vi "Settings Dialog.vi"(8 "error in (no error)":errorcluster, 11 "Settings in":T5={"Acquisition"={"State"=enum."Idle S3DK", "Settings"="", "Online"=FALSE, "S3DK"={"Signals"={"Phasor"=[], "Analog"=[], "Digital"=[]}}, "CSV"={"CSV Path"=path "", "Index"=0, "Parcel Length"=0, "EOF?"=FALSE}}, "Logging"={"Logging State"=enum."Idle", "Settings"="", "Buffer"={"Index"=0, "Size"=15000, "Samples"=0, "Ordered ?"=FALSE}}, "Processing"={"Settings"="Processing", "Params Energy"={"Index"=0, "Size"=0, "Samples"=0, "Ordered ?"=FALSE}, "Refresh Rate"=0, "Filters Instances"=[], "Levels"={"Low"=0, "High"=0, "Danger"=0}, "Params PSD"={"Index"=0, "Size"=0, "Samples"=0, "Ordered ?"=FALSE}, "PSD Instances"=[], "Filter Config"=[], "PSDs"=[]}} {"Processing"."PSD Instances"."Averaging"."averaging mode" items=["No averaging", "RMS averaging", "Peak hold"]; "Processing"."PSD Instances"."Averaging"."weighting mode" items=["Linear", "Exponential"]; "Processing"."PSD Instances"."AR"."Method" items=["Forward-Backward", "Least-Squares", "Yule-Walker", "Burg-Lattice", "Geometric-Lattice"]; "Processing"."PSD Instances"."Welch"."window info"."window" items=["None ", "Hanning", "Hamming", "Blackman-Harris", "Exact Blackman", "Blackman", "Flat Top", "4 Term B-Harris ", "7 Term B-Harris", "Low Sidelobe"]; "Processing"."Filters Instances"."PSD Filter"."Forward Coefficients" format="%.4f"; "Processing"."Filters Instances"."PSD Filter"."Reverse Coefficients" format="%.4f"}) -> (0 "error out":errorcluster, 1 "Changed?":bool, 2 "UI Refresh Needed?":bool, 3 "Settings out":T5={"Acquisition"={"State"=enum."Idle S3DK", "Settings"="", "Online"=FALSE, "S3DK"={"Signals"={"Phasor"=[], "Analog"=[], "Digital"=[]}}, "CSV"={"CSV Path"=path "", "Index"=0, "Parcel Length"=0, "EOF?"=FALSE}}, "Logging"={"Logging State"=enum."Idle", "Settings"="", "Buffer"={"Index"=0, "Size"=15000, "Samples"=0, "Ordered ?"=FALSE}}, "Processing"={"Settings"="Processing", "Params Energy"={"Index"=0, "Size"=0, "Samples"=0, "Ordered ?"=FALSE}, "Refresh Rate"=0, "Filters Instances"=[], "Levels"={"Low"=0, "High"=0, "Danger"=0}, "Params PSD"={"Index"=0, "Size"=0, "Samples"=0, "Ordered ?"=FALSE}, "PSD Instances"=[], "Filter Config"=[], "PSDs"=[]}} {"Processing"."PSD Instances"."Averaging"."averaging mode" items=["No averaging", "RMS averaging", "Peak hold"]; "Processing"."PSD Instances"."Averaging"."weighting mode" items=["Linear", "Exponential"]; "Processing"."PSD Instances"."AR"."Method" items=["Forward-Backward", "Least-Squares", "Yule-Walker", "Burg-Lattice", "Geometric-Lattice"]; "Processing"."PSD Instances"."Welch"."window info"."window" items=["None ", "Hanning", "Hamming", "Blackman-Harris", "Exact Blackman", "Blackman", "Flat Top", "4 Term B-Harris ", "7 Term B-Harris", "Low Sidelobe"]; "Processing"."Filters Instances"."PSD Filter"."Forward Coefficients" format="%.4f"; "Processing"."Filters Instances"."PSD Filter"."Reverse Coefficients" format="%.4f"})   [LabVIEW 2017, in "Settings.lvlib"]
doc: "Dialog for selecting user specified settings."
uses:
  Settings.lvlib
  Settings.ctl
  acquisition/Acquisition Settings.ctl
  acquisition/Acquisition State.ctl
  logging/Logging Configuration.ctl
  logging/Logging State.ctl
  libs/PMU Buffer/Buffer Settings.ctl
  processing/Processing Settings.ctl
  processing/Filters.ctl
  processing/Levels.ctl
  processing/PSD Setting.ctl
  processing/BP Filter Settings.ctl
  <vilib>/Analysis/3filter.llb/Filter Passband Type.ctl
  acquisition/Acquisition.lvlib
  logging/Logging.lvlib
  processing/Processing.lvlib
  libs/PMU Buffer/PMU data buffer.lvlib
  <vilib>/Analysis/NI_AALBase.lvlib
panel:
  in  "Levels":T1
  in  "Tab Control":T2(tab)
  in  "Set 1":T3 {"Averaging"."Nb" min=1; "Averaging"."Weighting Mode" items=["Linear", "Exponential"]; "Averaging"."Averaging Mode" items=["No averaging", "RMS averaging", "Peak hold"]; "Welch"."window info"."window" items=["None ", "Hanning", "Hamming", "Blackman-Harris", "Exact Blackman", "Blackman", "Flat Top", "4 Term B-Harris ", "7 Term B-Harris", "Low Sidelobe"]; "AR"."Method" items=["Forward-Backward", "Least-Squares", "Yule-Walker", "Burg-Lattice", "Geometric-Lattice"]}
  in  "Set 1":T4={"Type"=enum."Bandpass", "Freq low"=0.11, "Freq high"=1.0, "Filter Order"=11} {"Filter Order" min=2 max=15 scale=7.0..15.0}
  in  "Set 2":T4={"Type"=enum."Bandpass", "Freq low"=0.11, "Freq high"=1.0, "Filter Order"=11} {"Filter Order" min=2 max=15 scale=7.0..15.0}
  in  "Set 2":T3 {"Averaging"."Nb" min=1; "Averaging"."Weighting Mode" items=["Linear", "Exponential"]; "Averaging"."Averaging Mode" items=["No averaging", "RMS averaging", "Peak hold"]; "Welch"."window info"."window" items=["None ", "Hanning", "Hamming", "Blackman-Harris", "Exact Blackman", "Blackman", "Flat Top", "4 Term B-Harris ", "7 Term B-Harris", "Low Sidelobe"]; "AR"."Method" items=["Forward-Backward", "Least-Squares", "Yule-Walker", "Burg-Lattice", "Geometric-Lattice"]}
  in  "Set 3":T4={"Type"=enum."Bandpass", "Freq low"=0.11, "Freq high"=1.0, "Filter Order"=11} {"Filter Order" min=2 max=15 scale=7.0..15.0}
  in  "Set 3":T3 {"Averaging"."Nb" min=1; "Averaging"."Weighting Mode" items=["Linear", "Exponential"]; "Averaging"."Averaging Mode" items=["No averaging", "RMS averaging", "Peak hold"]; "Welch"."window info"."window" items=["None ", "Hanning", "Hamming", "Blackman-Harris", "Exact Blackman", "Blackman", "Flat Top", "4 Term B-Harris ", "7 Term B-Harris", "Low Sidelobe"]; "AR"."Method" items=["Forward-Backward", "Least-Squares", "Yule-Walker", "Burg-Lattice", "Geometric-Lattice"]}
  in  "Set 4":T4={"Type"=enum."Bandpass", "Freq low"=0.11, "Freq high"=1.0, "Filter Order"=11} {"Filter Order" min=2 max=15 scale=7.0..15.0}
  in  "Set 4":T3 {"Averaging"."Nb" min=1; "Averaging"."Weighting Mode" items=["Linear", "Exponential"]; "Averaging"."Averaging Mode" items=["No averaging", "RMS averaging", "Peak hold"]; "Welch"."window info"."window" items=["None ", "Hanning", "Hamming", "Blackman-Harris", "Exact Blackman", "Blackman", "Flat Top", "4 Term B-Harris ", "7 Term B-Harris", "Low Sidelobe"]; "AR"."Method" items=["Forward-Backward", "Least-Squares", "Yule-Walker", "Burg-Lattice", "Geometric-Lattice"]}
  in  "Online?":bool
  in  "Parcel Length":i32
  in  "Path":path
  in  "Refresh Rate":u32(ring) caption="Hz" items=["1"=1000, "5"=200, "10"=100, "25"=40, "50"=20]
  in  "Buffer Size":i32
  in  "Cancel Button":bool
  in  "OK Button":bool
  # "Non visible portion of dialog (needed for connector pane)."
  # "Welch Parameter"
  # "AR Spectrum"
  # "Welch Parameter"
  # "AR Spectrum"
  # "Welch Parameter"
  # "AR Spectrum"
  # "Welch Parameter"
  # "AR Spectrum"
  # "Buffer Paremeters"
  # "Buffer Paremeters"
  # "Buffer Paremeters"
  # "Buffer Paremeters"
  # "Buffer Paremeters"
  # "Buffer Paremeters"
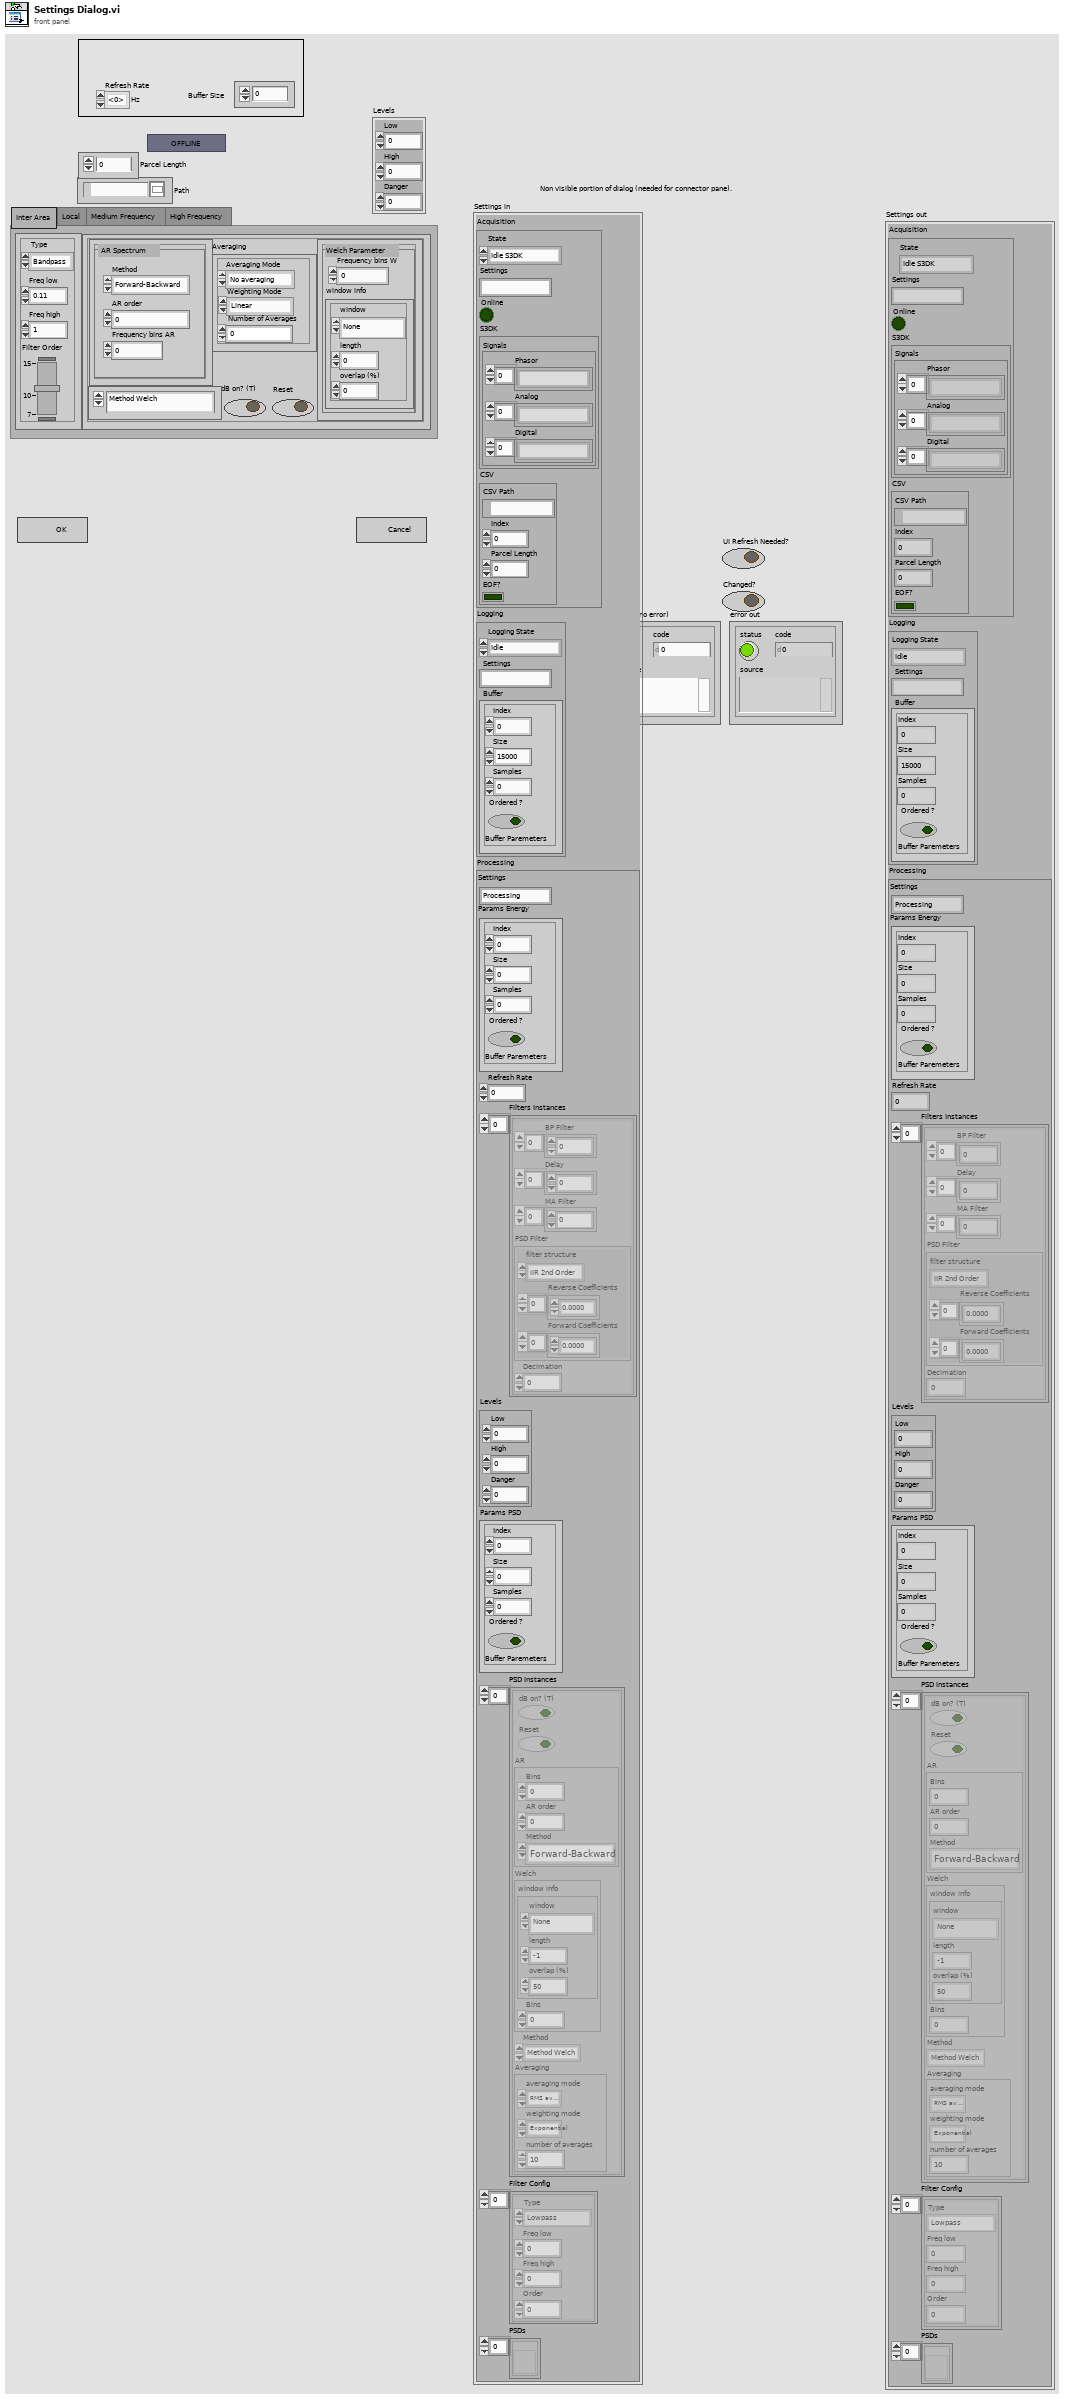
[diagram p1: front panel]
types:
  T1 = typedef "Processing.lvlib/Levels.ctl" = cluster{"Low":i32, "High":i32, "Danger":i32}
  T2 = enum32{"Inter Area", "Local", "Medium Frequency", "High Frequency"}
  T3 = cluster{"dB on? (T)":bool, "Reset":bool, "AR":cluster{"Bins":i32, "Method":u16, "AR order":i32}, "Welch":cluster{"window info":cluster{"window":u16, "length":i32, "overlap (%)":dbl}, "Bins":i32}, "Method":enum16{"Method Welch", "Method AR", "Both"}, "Averaging":cluster{"Averaging Mode":u16, "Weighting Mode":u16, "Nb":u32}}
  T4 = cluster{"Type":enum16{"Lowpass", "Highpass", "Bandpass", "Bandstop"}, "Freq low":dbl, "Freq high":dbl, "Filter Order":i32}
  T5 = typedef "Settings.lvlib/Settings.ctl" = cluster{"Acquisition":T6, "Logging":T8, "Processing":T11}
  T6 = typedef "Acquisition.lvlib/Acquisition Settings.ctl" = cluster{"State":T7, "Settings":string, "Online":bool, "S3DK":cluster{"Signals":cluster{"Phasor":string[], "Analog":string[], "Digital":string[]}}, "CSV":cluster{"CSV Path":path, "Index":i32, "Parcel Length":i32, "EOF?":bool}}
  T7 = typedef "Acquisition.lvlib/Acquisition State.ctl" = enum16{"Idle", "Idle S3DK", "Acquiring S3DK", "Idle CSV", "Acquiring CSV"}
  T8 = typedef "Logging.lvlib/Logging Configuration.ctl" = cluster{"Logging State":T9, "Settings":string, "Buffer":T10}
  T9 = typedef "Logging.lvlib/Logging State.ctl" = enum16{"Idle", "Logging"}
  T10 = typedef "PMU data buffer.lvlib/Buffer Settings.ctl" = cluster{"Index":i32, "Size":i32, "Samples":i32, "Ordered ?":bool}
  T11 = typedef "Processing.lvlib/Processing Settings.ctl" = cluster{"Settings":string, "Params Energy":T10, "Refresh Rate":u32, "Filters Instances":T12[], "Levels":T1, "Params PSD":T10, "PSD Instances":T13[], "Filter Config":T14[], "PSDs":refnum<vi>[]}
  T12 = typedef "Processing.lvlib/Filters.ctl" = cluster{"BP Filter":dbl[], "Delay":dbl[], "MA Filter":dbl[], "PSD Filter":cluster{"filter structure":enum32{"IIR 2nd Order", "IIR 4th Order"}, "Reverse Coefficients":dbl[], "Forward Coefficients":dbl[]}, "Decimation":i32}
  T13 = typedef "Processing.lvlib/PSD Setting.ctl" = cluster{"dB on? (T)":bool, "Reset":bool, "AR":cluster{"Bins":i32, "AR order":i32, "Method":u16}, "Welch":cluster{"window info":cluster{"window":u16, "length":i32, "overlap (%)":dbl}, "Bins":i32}, "Method":enum16{"Method Welch", "Method AR", "Both"}, "Averaging":cluster{"averaging mode":u16, "weighting mode":u16, "number of averages":u32}}
  T14 = typedef "Processing.lvlib/BP Filter Settings.ctl" = cluster{"Type":T15, "Freq low":dbl, "Freq high":dbl, "Order":i32}
  T15 = typedef "NI_AALBase.lvlib/Filter Passband Type.ctl" = enum32{"Lowpass", "Highpass", "Bandpass", "Bandstop"}
  T16 = cluster{"dB on? (T)":bool, "Reset":bool, "AR":cluster{"Bins":i32, "Method":u16, "AR order":i32}, "Welch":cluster{"window info":cluster{"window":u16, "length":i32, "overlap (%)":dbl}, "Bins":i32}, "Method":enum16{"Method Welch", "Method AR", "Both"}, "Averaging":cluster{"Averaging Mode":u16, "Weighting Mode":u16, "Nb":u32}}[]
  T17 = cluster{"Type":enum16{"Lowpass", "Highpass", "Bandpass", "Bandstop"}, "Freq low":dbl, "Freq high":dbl, "Filter Order":i32}[]
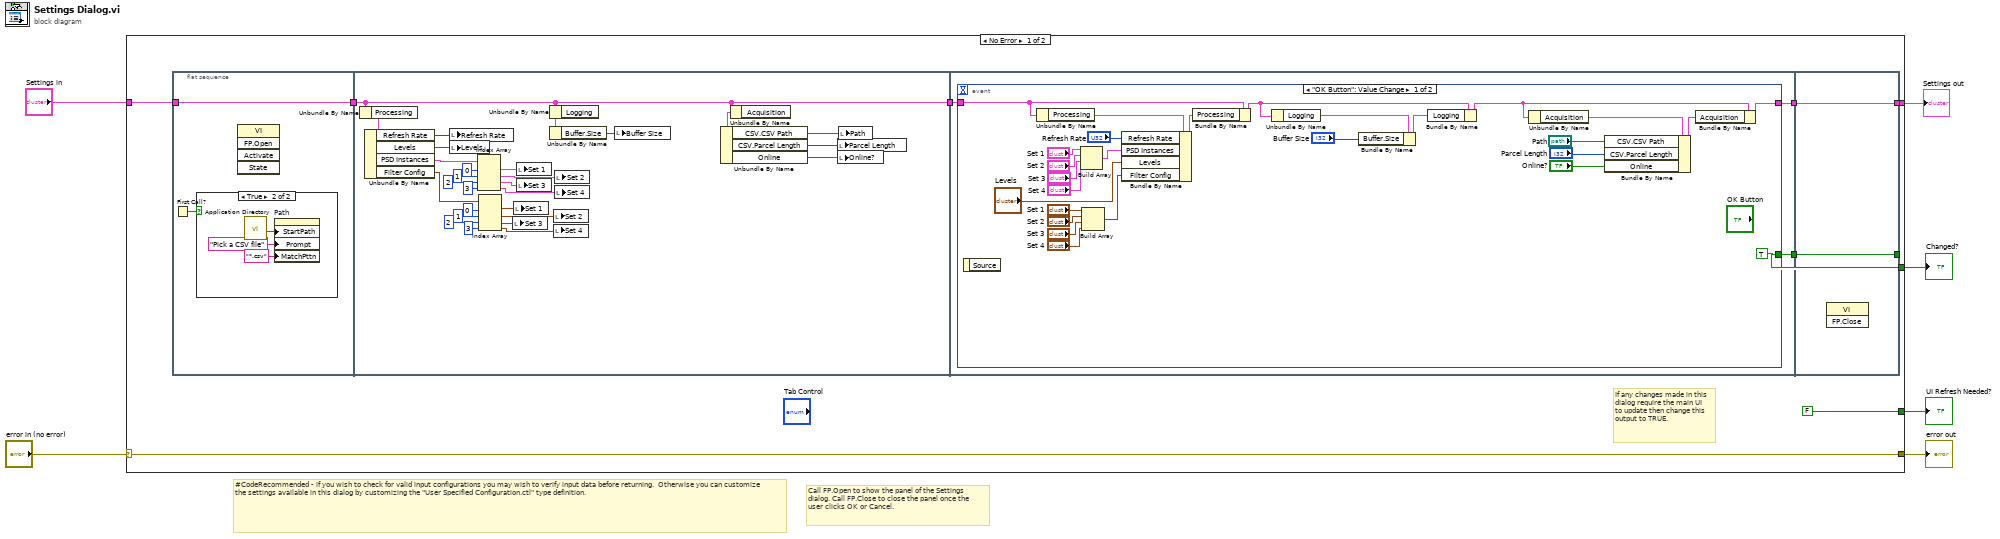
[diagram p0: block diagram]
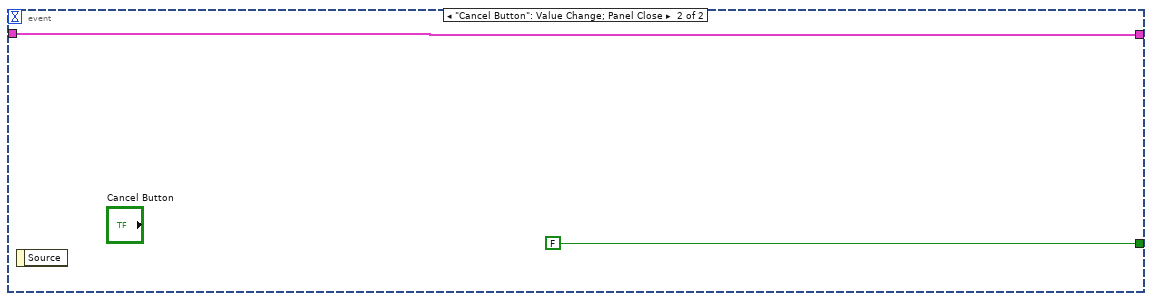
[diagram p3: hidden frame]
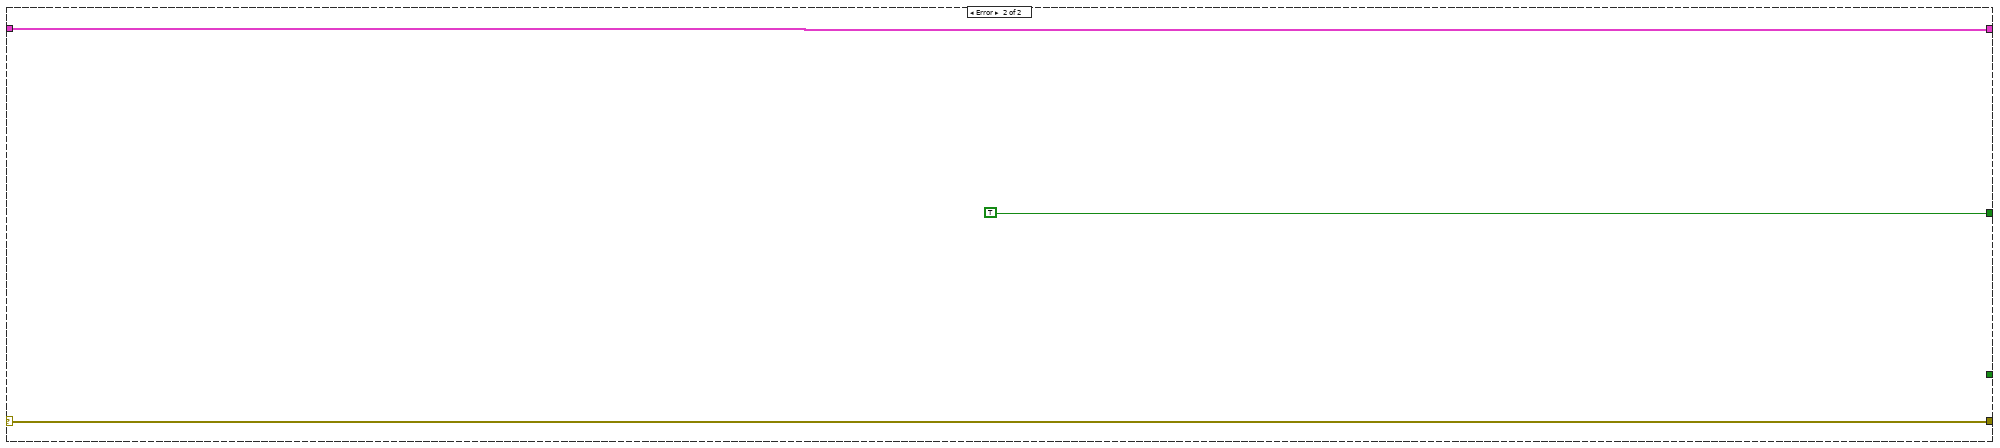
[diagram p4: hidden frame]
diagram:
  # "Call FP.Open to show the panel of the Settings dialog. Call FP.Close to close the panel once the user clicks OK or Cancel."
  # "#CodeRecommended - if you wish to check for valid input configurations you may wish to verify input data before returning.  Otherwise you can customize the settings available in this dialog by customizing the \"User Specified Configuration.ctl\" type definition."
  n1 = case shown="No Error" "error in (no error)" {
    selector: "error in (no error)" -> [w15 w85]
    tunnel: [w15 w85] -> w5
    tunnel: "Settings in" -> [w11 w84]
    tunnel: [w12 w84] -> w3
    tunnel: [FALSE ("UI Refresh Needed?") _] -> w2
    tunnel: [w13 TRUE ("UI Refresh Needed?")] -> w1
    frame No Error {
      # "If any changes made in this dialog require the main UI to update then change this output to TRUE."
      n2 = flat-sequence {
        tunnel: w11 -> [w17]
        tunnel: [w17] -> w8
        tunnel: w8 -> [w43]
        tunnel: [w43] -> w7
        tunnel: w7 -> [w49]
        tunnel: [w51] -> w10
        tunnel: [w50] -> w9
        tunnel: [w81] -> w12
        tunnel: [w82] -> w13
        tunnel: w10 -> [w82]
        tunnel: w9 -> [w81]
        frame #0 {
          n3 = First Call?() -> (First Call?: T/F=w16:bool)
          n4 = case shown="True" w16 {
            frame False {
            }
            frame True {
              n5 = call <vilib>:"Application Directory.vi"() -> ("Application Directory"=w20:path)
              n6 = property on="Path" class="Path"("StartPath"=w20, "Prompt"="Pick a CSV file" ("Browse Options:Prompt"), "MatchPttn"="*.csv" ("Browse Options:Match Pattern")) -> ()  [unwired: 2 in, 2 out]
            }
          }
          n7 = invoke class="VI" method="FP.Open"() -> ()  [unwired: 5 in, 5 out]
        }
        frame #1 {
          n8 = Unbundle By Name(w43) -> ("Processing"=w48:T11)
          n9 = Unbundle By Name(w48) -> ("Refresh Rate"=w45:u32, "Levels"=w39:T1, "PSD Instances"=w38:T13[], "Filter Config"=w25:T14[])
          n10 = local write "Refresh Rate"(w45) -> ()
          n11 = local write "Levels"(w39) -> ()
          n12 = Index Array(array=w38, index #1=0 ("index"), index #2=1 ("index"), index #3=2 ("index"), index #4=3 ("index")) -> (element #1=w33:T13, element #2=w32:T13, element #3=w31:T13, element #4=w30:T13)
          n13 = Index Array(array=w25, index #1=0 ("index"), index #2=1 ("index"), index #3=2 ("index"), index #4=3 ("index")) -> (element #1=w24:T14, element #2=w23:T14, element #3=w22:T14, element #4=w21:T14)
          n14 = local write "Set 3"(w22) -> ()
          n15 = local write "Set 1"(w24) -> ()
          n16 = local write "Set 1"(w33) -> ()
          n17 = local write "Set 3"(w31) -> ()
          n18 = Unbundle By Name(w43) -> ("Logging"=w47:T8)
          n19 = Unbundle By Name(w47) -> ("Buffer.Size"=w46:i32)
          n20 = local write "Set 2"(w23) -> ()
          n21 = local write "Set 4"(w21) -> ()
          n22 = local write "Set 2"(w32) -> ()
          n23 = local write "Set 4"(w30) -> ()
          n24 = local write "Buffer Size"(w46) -> ()
          n25 = Unbundle By Name(w43) -> ("Acquisition"=w44:T6)
          n26 = Unbundle By Name(w44) -> ("CSV.CSV Path"=w42:path, "CSV.Parcel Length"=w41:i32, "Online"=w40:bool)
          n27 = local write "Parcel Length"(w41) -> ()
          n28 = local write "Online?"(w40) -> ()
          n29 = local write "Path"(w42) -> ()
        }
        frame #2 {
          n30 = event shown="[0] \"OK Button\": Value Change" {
            selector: _ -> [_ _]
            dyn-events: _ -> [_ _]
            timeout: _ -> [_ _]
            tunnel: [w64 w80] -> w50
            tunnel: w49 -> [w75 w80]
            tunnel: [TRUE ("UI Refresh Needed?") FALSE ("UI Refresh Needed?")] -> w51
            event "OK Button": Value Change {
              n31 = event-data() -> ()  [unwired: 1 in, 1 out]
              n32 = Unbundle By Name(w75) -> ("Processing"=w77:T11)
              n33 = Build Array("Set 1", "Set 2", "Set 3", "Set 4") -> (w58:T16)
              n34 = Build Array("Set 1", "Set 2", "Set 3", "Set 4") -> (w52:T17)
              n35 = Bundle By Name(cluster=w77, "Refresh Rate"="Refresh Rate", "PSD Instances"=w58, "Levels"="Levels", "Filter Config"=w52) -> (w76:T11)
              n36 = Bundle By Name(cluster=w75, "Processing"=w76) -> (w69:T5)
              n37 = Unbundle By Name(w69) -> ("Logging"=w72:T8)
              n38 = Bundle By Name(cluster=w72, "Buffer.Size"="Buffer Size") -> (w73:T8)
              n39 = Bundle By Name(cluster=w69, "Logging"=w73) -> (w67:T5)
              n40 = Unbundle By Name(w67) -> ("Acquisition"=w71:T6)
              n41 = Bundle By Name(cluster=w71, "CSV.CSV Path"="Path", "CSV.Parcel Length"="Parcel Length", "Online"="Online?") -> (w70:T6)
              n42 = Bundle By Name(cluster=w67, "Acquisition"=w70) -> (w64:T5)
            }
            event "Cancel Button": Value Change; Panel Close {
              n43 = event-data() -> ()  [unwired: 1 in, 1 out]
            }
          }
        }
        frame #3 {
          n44 = invoke class="VI" method="FP.Close"() -> ()  [unwired: 3 in, 3 out]
        }
      }
    }
    frame Error {
    }
  }
  "UI Refresh Needed?" <- w2
  "error out" <- w5
  "Settings out" <- w3
  "Changed?" <- w1
